vi "Example Graph.vi"() -> ()   [LabVIEW 2010]
uses:
  C:/tf/play/labview/Tinkerforge.dll
panel:
  in  "stop":bool
  out "graph":sgl[](graph)
  in  "uid":string="dg7"
  in  "port":i32=4223
  in  "host":string="localhost"
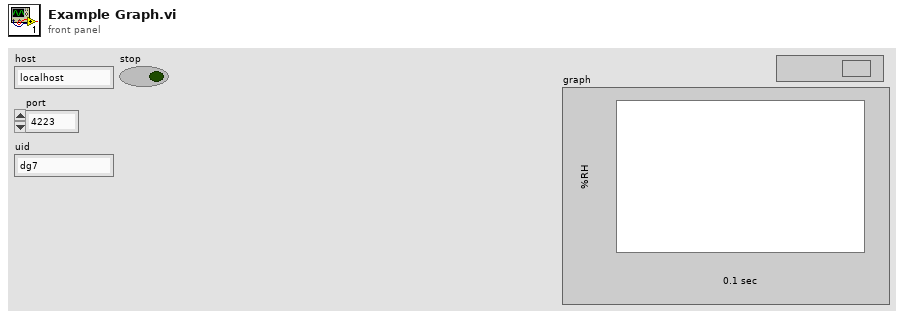
[diagram p1: front panel]
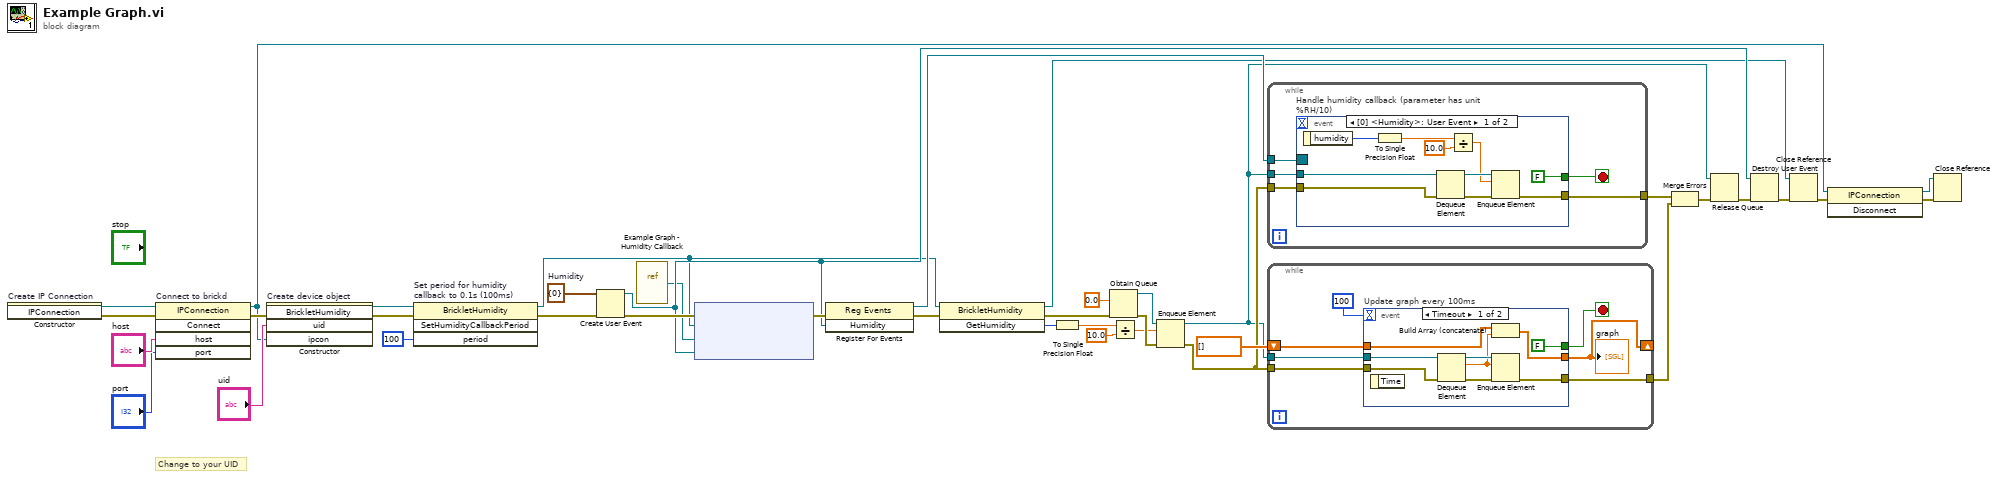
[diagram p0: block diagram]
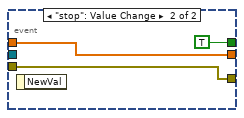
[diagram p2: hidden frame]
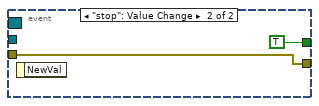
[diagram p3: hidden frame]
diagram:
  w25 = cluster{"humidity":i32} {"humidity"=0}  # Humidity
  # "Change to your UID"
  n1 = constructor on="Create IP Connection" class="IPConnection"() -> (reference out=w39:refnum<k24>, error out=w10:errorcluster)  [unwired: 3 in, 1 out]
  n2 = invoke on="Connect to brickd" class="IPConnection" method="Connect"(reference=w39, error in=w10, "host"="host", "port"="port") -> (reference out=w32:refnum<k24>, error out=w35:errorcluster)  [unwired: 1 in, 3 out]
  n3 = constructor on="Create device object" class="BrickletHumidity"(error in=w35, "uid"="uid", "ipcon"=w32) -> (reference out=w22:refnum<k24>, error out=w24:errorcluster)  [unwired: 2 in, 3 out]
  n4 = invoke on="Set period for humidity\ncallback to 0.1s (100ms)" class="BrickletHumidity" method="SetHumidityCallbackPeriod"(reference=w22, error in=w24, "period"=i64 100) -> (reference out=w2:refnum<k24>, error out=w23:errorcluster)  [unwired: 1 in, 2 out]
  n5 = Create User Event(user event datatype=w25, error in=w23) -> (user event=w27:refnum<user-event>, error out=w30:errorcluster)
  n6 = vi-ref "Example Graph - Humidity Callback.vi"() -> ("vi reference"=w9:refnum<vi>)
  n7 = node ("Register Event Callback")(w30, w2, w9, w27) -> (w29:errorcluster)  [unwired: 1 in, 1 out]
  n8 = register-events(error in=w29, w27) -> (reference out=w28:refnum<event-registration>, error out=w8:errorcluster)  [unwired: 1 in]
  n9 = invoke class="BrickletHumidity" method="GetHumidity"(reference=w2, error in=w8) -> (reference out=w1:refnum<k24>, error out=w7:errorcluster, "GetHumidity"=w3:i32)  [unwired: 1 in]
  n10 = To Single Precision Float(number=w3) -> (single precision float=w5:sgl)
  n11 = Obtain Queue(element data type=sgl 0.0, error in (no error)=w7) -> (queue out=w14:refnum<queue>, error out=w16:errorcluster)  [unwired: 3 in, 1 out]
  n12 = Divide(x=w5, y=sgl 10.0) -> (x/y=w4:sgl)
  n13 = Enqueue Element(queue=w14, element=w4, error in (no error)=w16) -> (queue out=w11:refnum<queue>, error out=w15:errorcluster)  [unwired: 1 in, 1 out]
  n14 = while {
    tunnel: w28 -> [w44]
    tunnel: [w42] -> w19
    tunnel: w15 -> [w43]
    tunnel: w11 -> [w41]
    stop <- w40 stop-if-true
    n15 = event "Handle humidity callback (parameter has unit %RH/10)" shown="[0] <Humidity>: User Event" {
      selector: w44 -> [_ _]
      dyn-events: _ -> [_ _]
      timeout: _ -> [_ _]
      tunnel: w43 -> [w51 w55]
      tunnel: [w49 w55] -> w42
      tunnel: w41 -> [w48 _]
      tunnel: [FALSE TRUE] -> w40
      event User Event {
        n16 = event-data() -> ("humidity"=w52:i32)  [unwired: 1 in]
        n17 = To Single Precision Float(number=w52) -> (single precision float=w53:sgl)
        n18 = Dequeue Element(queue=w48, error in (no error)=w51) -> (queue out=w47:refnum<queue>, error out=w50:errorcluster)  [unwired: 1 in, 2 out]
        n19 = Divide(x=w53, y=sgl 10.0) -> (x/y=w46:sgl)
        n20 = Enqueue Element(queue=w47, element=w46, error in (no error)=w50) -> (error out=w49:errorcluster)  [unwired: 1 in, 2 out]
      }
      event "stop": Value Change {
        n21 = event-data() -> ()  [unwired: 1 in, 1 out]
      }
    }
  }
  n22 = while {
    tunnel: [w59] -> w20
    tunnel: w15 -> [w60]
    shift-right: [w61] -> _
    shift-left: sgl[] [] -> [w62]
    tunnel: w11 -> [w58]
    stop <- w57 stop-if-true
    n23 = event "Update graph every 100ms" shown="[0] Timeout" {
      selector: _ -> [_ _]
      dyn-events: _ -> [_ _]
      timeout: 100 -> [_ _]
      tunnel: [w72 w74] -> w61
      tunnel: w62 -> [w65 w74]
      tunnel: w60 -> [w71 w73]
      tunnel: [w68 w73] -> w59
      tunnel: w58 -> [w70 _]
      tunnel: [FALSE TRUE] -> w57
      event Timeout {
        n24 = event-data() -> ()  [unwired: 1 in, 1 out]
        n25 = Dequeue Element(queue=w70, error in (no error)=w71) -> (queue out=w67:refnum<queue>, element=w66:sgl, error out=w69:errorcluster)  [unwired: 1 in, 1 out]
        n26 = Build Array (concatenate)(w65, w66) -> (w72:sgl[])
        n27 = Enqueue Element(queue=w67, element=w66, error in (no error)=w69) -> (error out=w68:errorcluster)  [unwired: 1 in, 2 out]
      }
      event "stop": Value Change {
        n28 = event-data() -> ()  [unwired: 1 in, 1 out]
      }
    }
    "graph" <- w61
  }
  n29 = Merge Errors(w19, w20) -> (w13:errorcluster)
  n30 = Release Queue(queue=w11, error in (no error)=w13) -> (error out=w12:errorcluster)  [unwired: 1 in, 2 out]
  n31 = Destroy User Event(user event=w27, error in=w12) -> (error out=w26:errorcluster)
  n32 = Close Reference(reference=w1, error in (no error)=w26) -> (error out=w34:errorcluster)
  n33 = invoke class="IPConnection" method="Disconnect"(reference=w32, error in=w34) -> (reference out=w31:refnum<k24>, error out=w33:errorcluster)  [unwired: 1 in, 1 out]
  n34 = Close Reference(reference=w31, error in (no error)=w33) -> ()  [unwired: 1 out]
